vi "test1-ModuleCreatedDestroyed_Queue.vi"(8 "error in (no error)":errorcluster, 11 "TestCase in":refnum<class "testcase-CSMGlobalLog.lvclass">) -> (0 "error out":errorcluster, 3 "TestCase out":refnum<class "testcase-CSMGlobalLog.lvclass">)   [LabVIEW 2017, in "testcase-CSMGlobalLog.lvclass"]
uses:
  testcase-CSMGlobalLog.lvclass
  testcase-CSMGlobalLog.lvclass/testcase-CSMGlobalLog.ctl
  64b6e408-f0cd-4aee-a387-1a6bb95babb2.vi
  <vilib>/addons/_JKI Toolkits/VI Tester/TestCase.llb/TestCase.lvclass
  src/user.lib/_NEVSTOP/Communicable State Machine(CSM)/Utility/Periodic String Filter Setting.ctl
  src/user.lib/_NEVSTOP/Communicable State Machine(CSM)/Communicable State Machine.lvlib
  CSM/CSM-Testcase.lvlib
  C:/Program Files (x86)/National Instruments/LabVIEW 2017/vi.lib/addons/_JKI Toolkits/VI Tester/TestCase.llb/TestCase.lvclass
panel:
  out "String Cache Each Loop":string
  out "String cache total":string
  out "LoopCount":i32
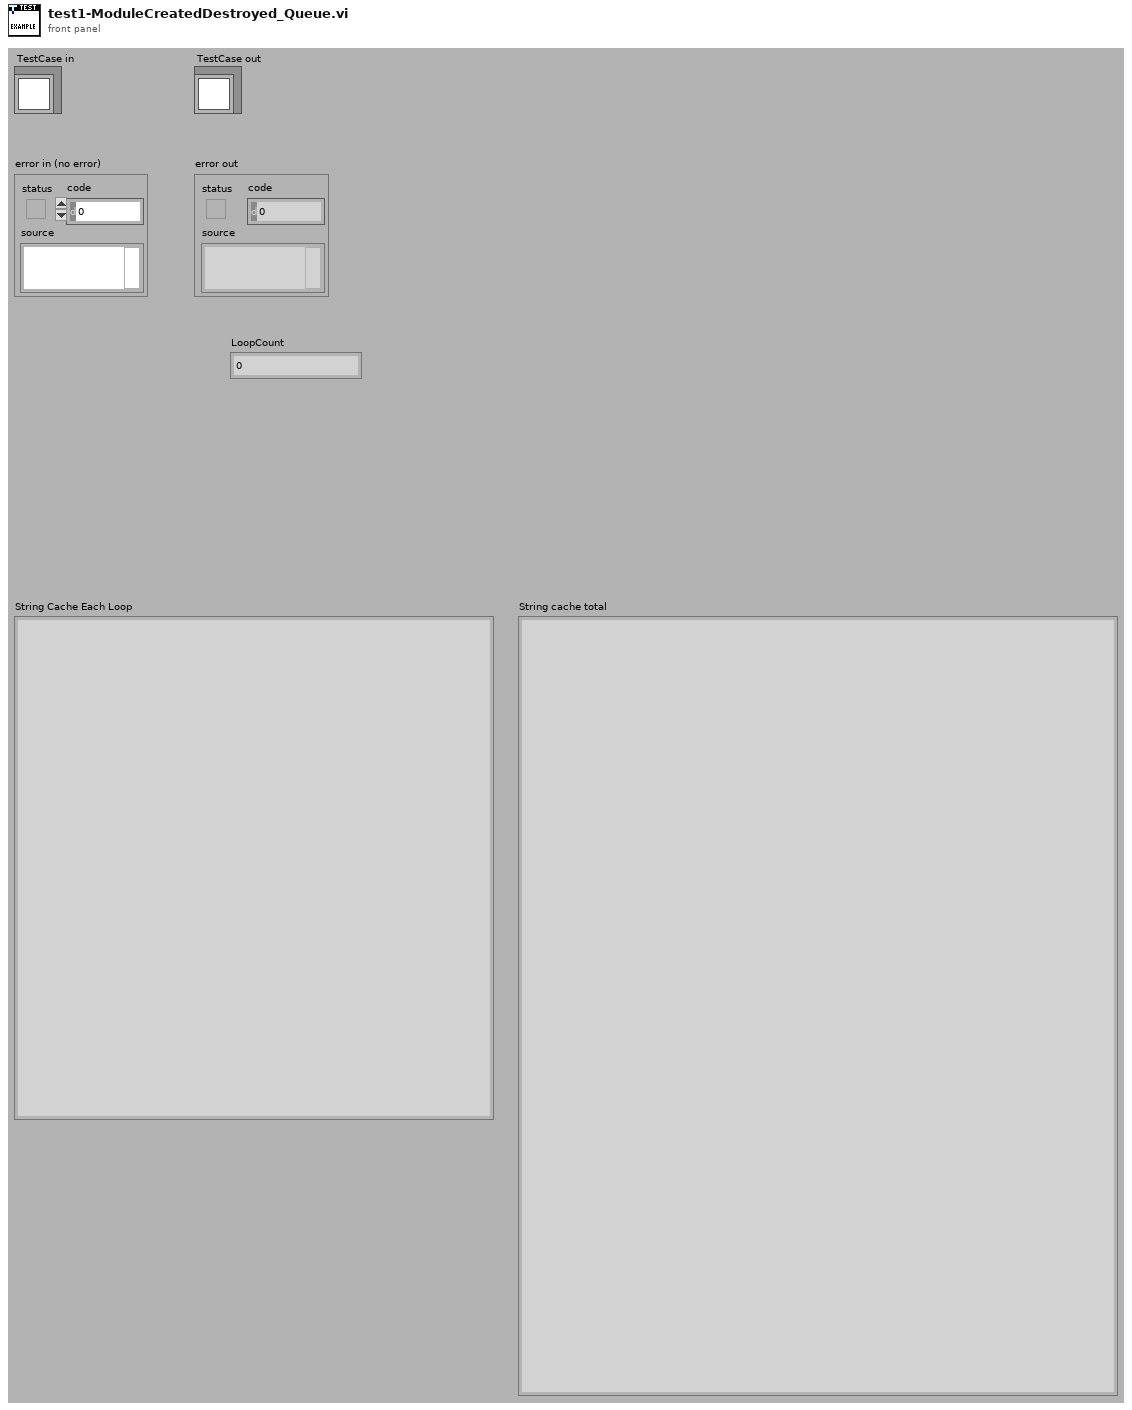
[diagram p1: front panel]
types:
  T1 = typedef "Communicable State Machine.lvlib/Periodic String Filter Setting.ctl" = cluster{"threashold(#/s)":dbl, "Check Peroid(s)":dbl}
  T2 = typedef "Communicable State Machine.lvlib/_CSM_GlobalLog_MSG.ctl" = cluster{"Name (\"\" to Use UUID)":string, "Current State":string, "Arguments":string, "Source Message":T3, "Source Module":string, "Complete(T)/Start(F)":bool, "LogType":T4, "Time Stamp":timestamp}
  T3 = typedef "Communicable State Machine.lvlib/_CSM_Response Source Message.ctl" = cluster{"‘State":string, "’Arguments":string, "’Error":errorcluster}
  T4 = typedef "Communicable State Machine.lvlib/_CSM_GlobalLog_MSG_TYPE.ctl" = enum16{"User Log", "State Change", "Status", "Interrupt", "Register", "Unregister", "Error Log", "Module Created", "Module Destroyed", "Async Message", "No-Rep Async Message", "Sync Message"}
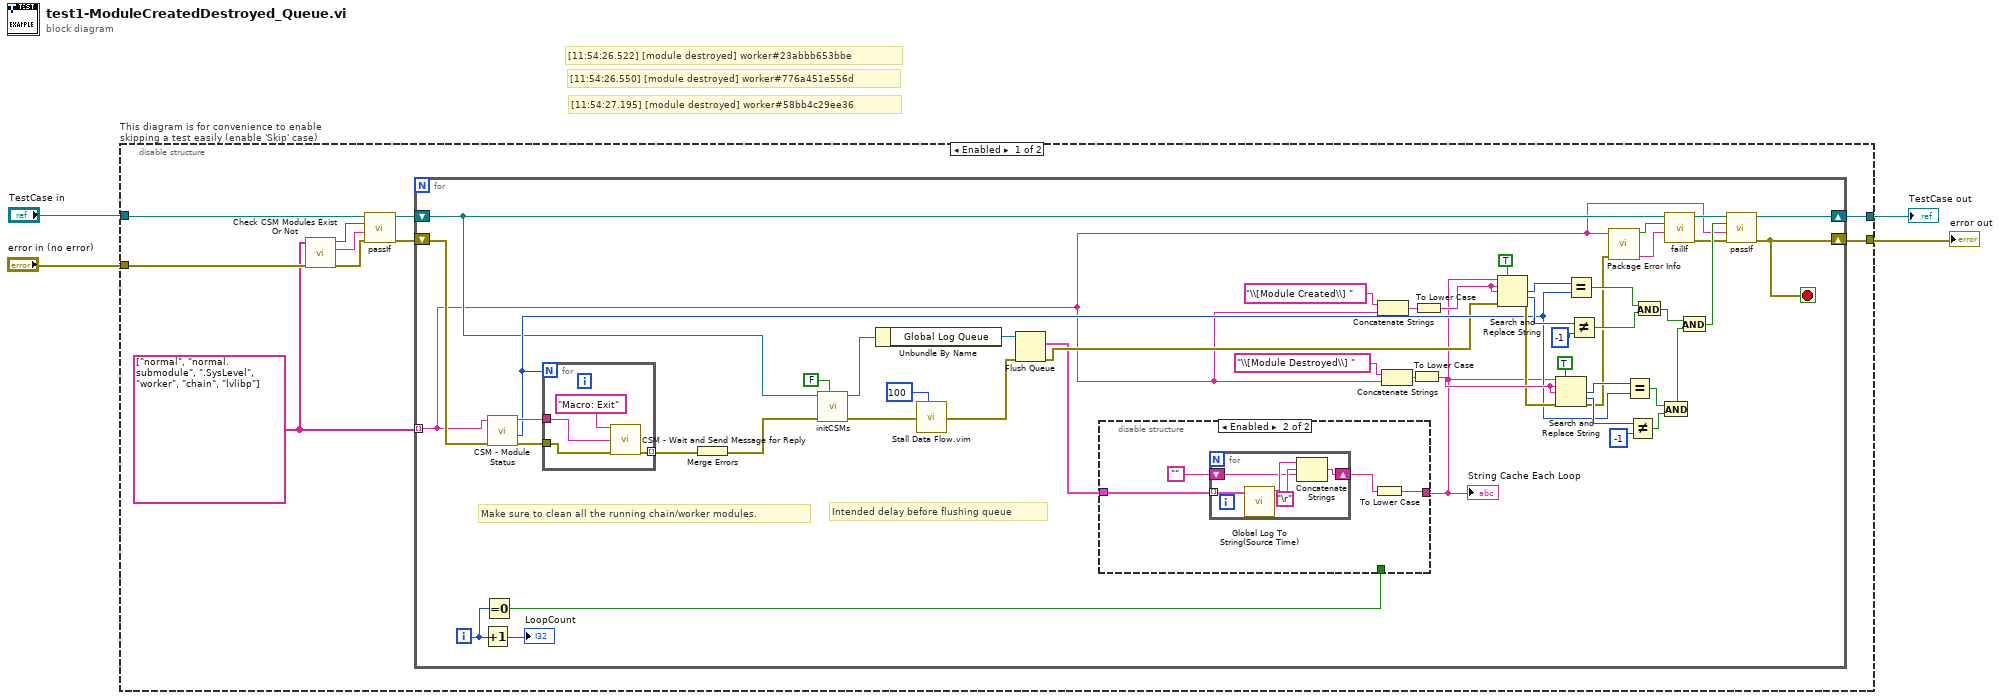
[diagram p0: block diagram]
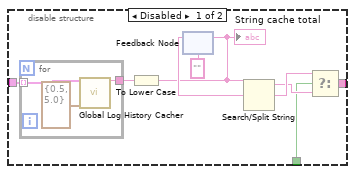
[diagram p2: hidden frame]
diagram:
  # "[11:54:26.522] [module destroyed] worker#23abbb653bbe"
  # "[11:54:27.195] [module destroyed] worker#58bb4c29ee36"
  # "[11:54:26.550] [module destroyed] worker#776a451e556d"
  n1 = disable-structure "This diagram is for convenience to enable skipping a test easily (enable 'Skip' case)" shown="Enabled" {
    disable-tunnel: "TestCase in" -> [w9 w92]
    disable-tunnel: [w13 w90] -> w1
    disable-tunnel: [w14 w91] -> w3
    disable-tunnel: "error in (no error)" -> [w7 w89]
    frame Enabled {
      w5 = string[] ["normal", "normal.submodule", ".SysLevel", "worker", "chain", "lvlibp"]
      n2 = call "Check CSM Modules Exist Or Not.vi"("error in"=w7, "CSM names in"=w5) -> ("error out"=w10:errorcluster, "Debug string"=w11:string, "All Modules Exist?"=w12:bool)  [unwired: 7 in]
      n3 = call-dynamic "passIf.vi"("error in (no error)"=w10, "message (\"\")"=w11, "pass"=w12, "TestCase in"=w9) -> ("error out"=w6:errorcluster, "TestCase out"=w8:refnum<class "testcase-CSMGlobalLog.lvclass">)  [unwired: 6 in]
      n4 = for {
        tunnel: w5 -> [w15] mode=indexing
        shift-right: [w31] -> w14
        shift-left: w6 -> [w23]
        shift-right: [w63] -> w13
        shift-left: w8 -> [w19]
        i -> [w25]
        stop <- w31 stop-if-true
        # "Intended delay before flushing queue"
        # "Make sure to clean all the running chain/worker modules."
        n5 = Increment(x=w25) -> (x+1=→"LoopCount":i32)
        n6 = Equal To 0?(x=w25) -> (x = 0?=w24:bool)
        n7 = call "CSM - Module Status.vi"("Error In"=w23, "CSM Name"=w15) -> ("error out"=w22:errorcluster, "#Nodes"=w38:i32, "CSM Name (Dup)"=w55:string)  [unwired: 5 in, 2 out]
        n8 = for {
          N: w38 -> [_]
          tunnel: [w87] -> w54 mode=indexing
          tunnel: w55 -> [w86]
          tunnel: w22 -> [w85]
          n9 = call "CSM - Wait and Send Message for Reply.vi"("State"="Macro: Exit", "Target Module"=w86, "Error In (No Error)"=w85) -> ("error out"=w87:errorcluster)  [unwired: 9 in, 3 out]
        }
        n10 = Merge Errors(w54) -> (w33:errorcluster)
        n11 = call "initCSMs.vi"("Enable building lvlibp?"=FALSE, "error in (no error)"=w33, "TestCase in"=w19) -> ("error out"=w30:errorcluster, "TestCase out"=w32:refnum<class "testcase-CSMGlobalLog.lvclass">)  [unwired: 7 in]
        n12 = Unbundle By Name(w32) -> ("Global Log Queue"=w62:refnum<queue>)
        n13 = call "Stall Data Flow.vim"("value in"=w30, "milliseconds to wait"=u32 100) -> ("value out"=w29:errorcluster)  [unwired: 1 out]
        n14 = Flush Queue(queue=w62, error in (no error)=w29) -> (remaining elements=w27:T2[], error out=w34:errorcluster)  [unwired: 1 out]
        n15 = disable-structure shown="Enabled" {
          disable-tunnel: [w66 w76] -> w26
          disable-tunnel: w24 -> [w65 _]
          disable-tunnel: w27 -> [w64 w78]
          frame Disabled {
            n16 = for {
              tunnel: w64 -> [w75] mode=indexing
              tunnel: [w74] -> w72
              n17 = call "Global Log History Cacher.vi"("Global Log Data"=w75, "Settings"=T1 {"threashold(#/s)"=0.5, "Check Peroid(s)"=5.0}) -> ("String Cache"=w74:string)  [unwired: 13 in]
            }
            n18 = To Lower Case(string=w72) -> (all lower case string=w67:string)
            "String cache total" <- w67
            n19 = feedback #1("") -> (w71:string)
            n20 = feedback-in #1(w67) -> ()
            n21 = Search/Split String(string=w67, search string/char (-)=w71) -> (substring before match=w68:string, match + rest of string=w69:string)  [unwired: 1 in, 1 out]
            n22 = Select(t=w69, s=w65, f=w68) -> (s? t:f=w66:string)
          }
          frame Enabled {
            n23 = for {
              tunnel: w78 -> [w84] mode=indexing
              shift-right: [w80] -> w77
              shift-left: "" -> [w81]
              n24 = call "Global Log To String(Source Time).vi"("Log"=w84) -> ("Log String"=w83:string)  [unwired: 9 in]
              n25 = Concatenate Strings(w83, "\r", w81) -> (w80:string)
            }
            n26 = To Lower Case(string=w77) -> (all lower case string=w76:string)
          }
        }
        "String Cache Each Loop" <- w26
        n27 = Concatenate Strings("\\[Module Created\\] " ("regular expression"), w15) -> (w56:string)
        n28 = Concatenate Strings("\\[Module Destroyed\\] " ("regular expression"), w15) -> (w58:string)
        n29 = To Lower Case(string=w58) -> (all lower case string=w40:string)
        n30 = To Lower Case(string=w56) -> (all lower case string=w52:string)
        n31 = Search and Replace String(replace all?=TRUE ("replace all? (F)"), input string=w26, search string=w52, replace string=w52, error in=w34) -> (number of replacements=w51:i32, offset past replacement=w50:i32, error out=w39:errorcluster)  [unwired: 3 in, 1 out]
        n32 = Search and Replace String(replace all?=TRUE ("replace all? (F)"), input string=w26, search string=w40, replace string=w40, error in=w39) -> (number of replacements=w42:i32, offset past replacement=w43:i32, error out=w16:errorcluster)  [unwired: 3 in, 1 out]
        n33 = Equal?(x=w51, y=w38) -> (x = y?=w48:bool)
        n34 = Not Equal?(x=w50, y=-1) -> (x != y?=w47:bool)
        n35 = call "Package Error Info.vi"("error in"=w16, "String in"=w15) -> ("packed error info out"=w20:string, "error status"=w21:bool)  [unwired: 8 in]
        n36 = Equal?(x=w42, y=w38) -> (x = y?=w45:bool)
        n37 = Not Equal?(x=w43, y=-1) -> (x != y?=w46:bool)
        n38 = And(x=w48, y=w47) -> (x .and. y?=w37:bool)
        n39 = And(x=w45, y=w46) -> (x .and. y?=w36:bool)
        n40 = call-dynamic "failIf.vi"("message (\"\")"=w20, "fail"=w21, "TestCase in"=w19) -> ("error out"=w17:errorcluster, "TestCase out"=w18:refnum<class "testcase-CSMGlobalLog.lvclass">)  [unwired: 7 in]
        n41 = And(x=w37, y=w36) -> (x .and. y?=w35:bool)
        n42 = call-dynamic "passIf.vi"("error in (no error)"=w17, "message (\"\")"=w15, "pass"=w35, "TestCase in"=w18) -> ("error out"=w31:errorcluster, "TestCase out"=w63:refnum<class "testcase-CSMGlobalLog.lvclass">)  [unwired: 6 in]
      }
    }
    frame Disabled {
      # "skip test result while test is under development"
      n43 = call <vilib>:"skip.vi"("error in (no error)"=w89, "TestCase in"=w92) -> ("error out"=w91:errorcluster, "TestCase out"=w90:refnum<class "testcase-CSMGlobalLog.lvclass">)  [unwired: 8 in]
    }
  }
  "error out" <- w3
  "TestCase out" <- w1
